vi "New GPS on GIC D.vi"(11 "GIC Input":T1={"     Use ?\nOff       On"=[FALSE, TRUE, FALSE, TRUE], "Mode:"=FALSE, "Extra Port"="", "Hokuyo Port"="COM7", "Tx Prop  Port"="COM6", "Compass Port"="", "GPS Port"="", "Num of WPs"=0, "WP Lats and Longs"={"WP Lats"=[], "WP Longs"=[]}, "Obst Lats and Longs"={"Obst Lats"=[], "Obst Longs"=[]}, "Parameters"=[], "GPS Data"=[], "Compass"=0.0, "LMS Vector"=[], "Vision Vector"=[], "Direction Cmd"=0.0, "Speed Cmd"=0.0, "WP Vector"=[], "WP Number"=0, "Extra"=0, "SW Map"=[], "Path Cluster"={"Path x node"=[], "Path y node"=[]}, "Sim Course"=[]} {"Obst Lats and Longs"."Obst Longs" format="%#_8g"; "Obst Lats and Longs"."Obst Lats" format="%#_8g"}) -> (3 "GIC Output":T1={"     Use ?\nOff       On"=[FALSE, TRUE, FALSE, TRUE], "Mode:"=FALSE, "Extra Port"="", "Hokuyo Port"="COM7", "Tx Prop  Port"="COM6", "Compass Port"="", "GPS Port"="", "Num of WPs"=0, "WP Lats and Longs"={"WP Lats"=[], "WP Longs"=[]}, "Obst Lats and Longs"={"Obst Lats"=[], "Obst Longs"=[]}, "Parameters"=[], "GPS Data"=[], "Compass"=0.0, "LMS Vector"=[], "Vision Vector"=[], "Direction Cmd"=0.0, "Speed Cmd"=0.0, "WP Vector"=[], "WP Number"=0, "Extra"=0, "SW Map"=[], "Path Cluster"={"Path x node"=[], "Path y node"=[]}, "Sim Course"=[]} {"Obst Lats and Longs"."Obst Longs" format="%#_8g"; "Obst Lats and Longs"."Obst Lats" format="%#_8g"})   [LabVIEW 2014]
panel:
  # "New GPS on GIC D"
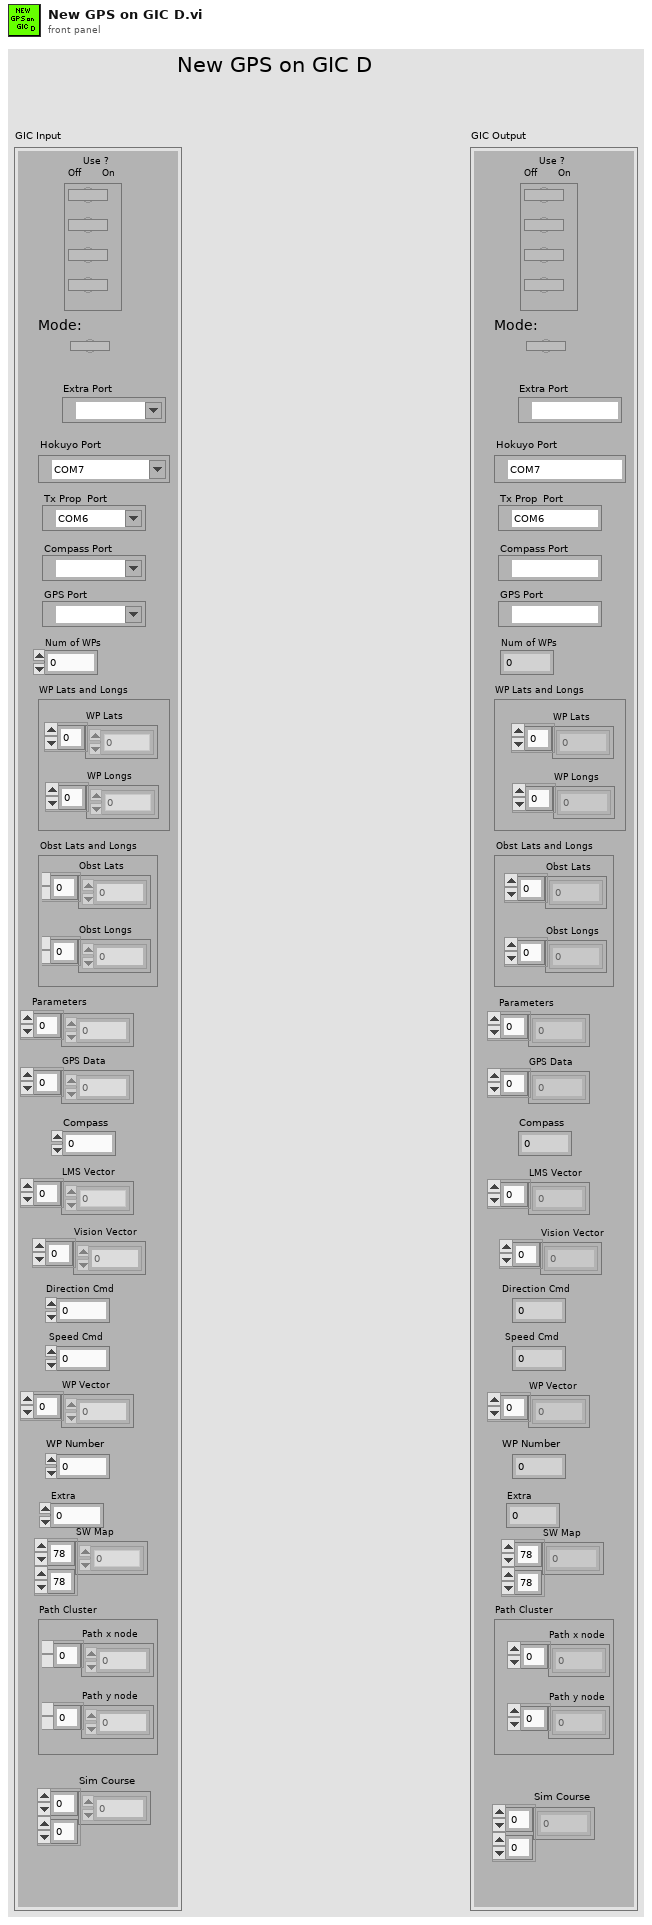
[diagram p1: front panel]
types:
  T1 = cluster{"     Use ?\nOff       On":bool[], "Mode:":bool, "Extra Port":refnum<visa-resource-name>, "Hokuyo Port":refnum<visa-resource-name>, "Tx Prop  Port":refnum<visa-resource-name>, "Compass Port":refnum<visa-resource-name>, "GPS Port":refnum<visa-resource-name>, "Num of WPs":i16, "WP Lats and Longs":cluster{"WP Lats":dbl[], "WP Longs":dbl[]}, "Obst Lats and Longs":cluster{"Obst Lats":dbl[], "Obst Longs":dbl[]}, "Parameters":dbl[], "GPS Data":dbl[], "Compass":dbl, "LMS Vector":dbl[], "Vision Vector":dbl[], "Direction Cmd":dbl, "Speed Cmd":dbl, "WP Vector":dbl[], "WP Number":i32, "Extra":i16, "SW Map":i32[][], "Path Cluster":cluster{"Path x node":dbl[], "Path y node":dbl[]}, "Sim Course":i8[][]}
  T2 = cluster{"     Use ?\nOff       On":bool[], "Mode:":bool, "Rx Prop Port":refnum<visa-resource-name>, "Hokuyo Port":refnum<visa-resource-name>, "Tx Prop  Port":refnum<visa-resource-name>, "Compass Port":refnum<visa-resource-name>, "GPS Port":refnum<visa-resource-name>, "Num of WPs":i16, "WP Lats and Longs":cluster{"WP Lats":dbl[], "WP Longs":dbl[]}, "Obst Lats and Longs":cluster{"Obst Lats":dbl[], "Obst Longs":dbl[]}, "Parameters":dbl[], "GPS Data":dbl[], "Compass":dbl, "LMS Vector":dbl[], "Vision Vector":dbl[], "Direction Cmd":dbl, "Speed Cmd":dbl, "WP Vector":dbl[], "WP Number":i32, "Extra":i16, "SW Map":i32[][], "Path Cluster":cluster{"Path x node":dbl[], "Path y node":dbl[]}, "Sim Course":i8[][]}
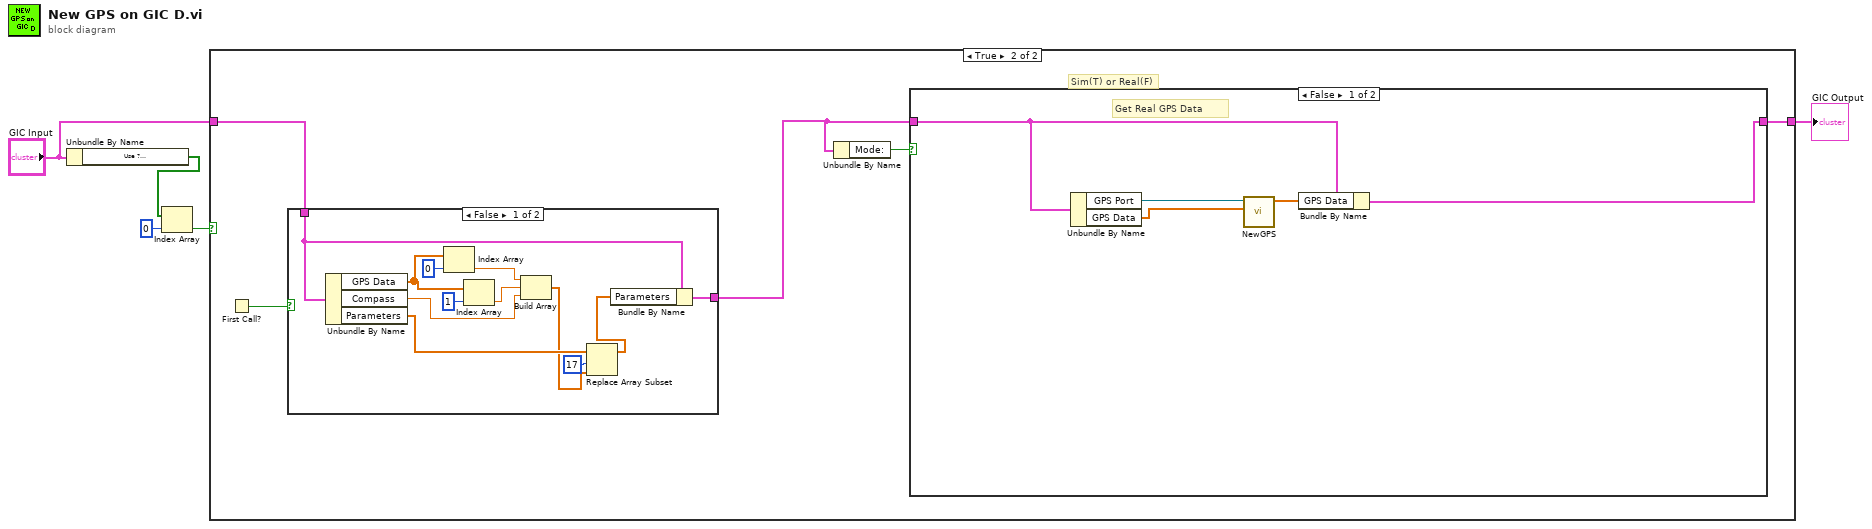
[diagram p0: block diagram]
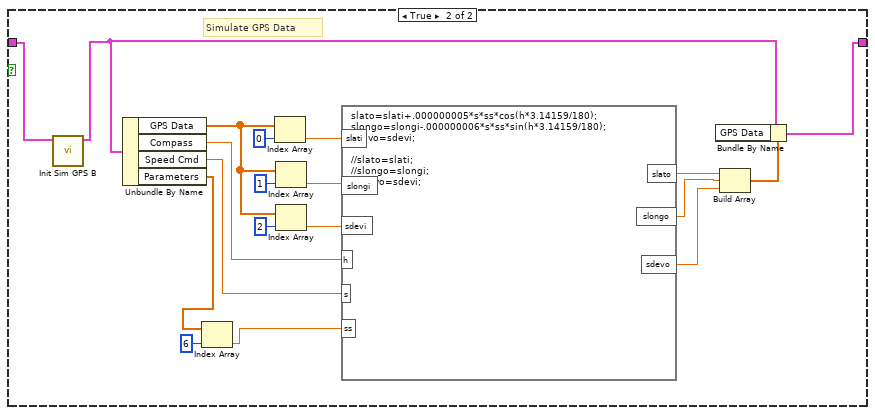
[diagram p4: hidden frame]
diagram:
  n1 = Unbundle By Name("GIC Input") -> ("Use ?\nOff       On"=w5:bool[])
  n2 = Index Array(array=w5, index=0) -> (element=w3:bool)
  n3 = case shown="True" w3 {
    tunnel: "GIC Input" -> [w6 w9]
    tunnel: [w6 w11] -> w1
    frame False {
    }
    frame True {
      # "Sim(T) or Real(F)"
      n4 = First Call?() -> (First Call?: T/F=w10:bool)
      n5 = case shown="False" w10 {
        tunnel: w9 -> [w12 w24]
        tunnel: [w13 w24] -> w8
        frame False {
          n6 = Unbundle By Name(w12) -> ("GPS Data"=w22:dbl[], "Compass"=w17:dbl, "Parameters"=w20:dbl[])
          n7 = Index Array(array=w22, index=0) -> (element=w19:dbl)
          n8 = Index Array(array=w22, index=1) -> (element=w18:dbl)
          n9 = Build Array(w19, w18, w17) -> (w15:dbl[])
          n10 = Replace Array Subset(array=w20, new element=w15, index=17) -> (w14:dbl[])
          n11 = Bundle By Name(cluster=w12, "Parameters"=w14) -> (w13:T1)
        }
        frame True {
        }
      }
      n12 = Unbundle By Name(w8) -> ("Mode:"=w7:bool)
      n13 = case shown="False" w7 {
        tunnel: w8 -> [w29 w30]
        tunnel: [w27 w35] -> w11
        frame False {
          # "Get Real GPS Data"
          n14 = Unbundle By Name(w29) -> ("GPS Port"=w26:refnum<visa-resource-name>, "GPS Data"=w25:dbl[])
          n15 = call "NewGPS.vi"("Input lat, long, dev"=w25, "GPS Com Port"=w26) -> ("Output lat, long, dev"=w28:dbl[])  [unwired: 9 in]
          n16 = Bundle By Name(cluster=w29, "GPS Data"=w28) -> (w27:T1)
        }
        frame True {
          # "Simulate GPS Data"
          n17 = call "Init Sim GPS B.vi"("GIC Input"=w30) -> ("GIC Output"=w34:T2)  [unwired: 10 in]
          n18 = Unbundle By Name(w34) -> ("GPS Data"=w44:dbl[], "Compass"=w41:dbl, "Speed Cmd"=w40:dbl, "Parameters"=w33:dbl[])
          n19 = Index Array(array=w33, index=6) -> (element=w31:dbl)
          n20 = Index Array(array=w44, index=0) -> (element=w48:dbl)
          n21 = Index Array(array=w44, index=1) -> (element=w46:dbl)
          n22 = Index Array(array=w44, index=2) -> (element=w43:dbl)
          n23 = formula code="slato=slati+.000000005*s*ss*cos(h*3.14159/180);\nslongo=slongi-.000000006*s*ss*sin(h*3.14159/180);\nsdevo=sdevi;\n\n//slato=slati;\n//slongo=slongi;\n//sdevo=sdevi;"("slati"=w48, "slongi"=w46, "sdevi"=w43, "h"=w41, "s"=w40, "ss"=w31) -> ("slato"=w39:dbl, "slongo"=w38:dbl, "sdevo"=w37:dbl)
          n24 = Build Array(w39, w38, w37) -> (w36:dbl[])
          n25 = Bundle By Name(cluster=w34, "GPS Data"=w36) -> (w35:T2)
        }
      }
    }
  }
  "GIC Output" <- w1
